vi "sub_DSP_main.vi"(8 "error in":errorcluster) -> (0 "error out":errorcluster)   [LabVIEW 2019]
uses:
  _ctrl/create-rw-close.ctl
  _ctrl/DSP_action.ctl
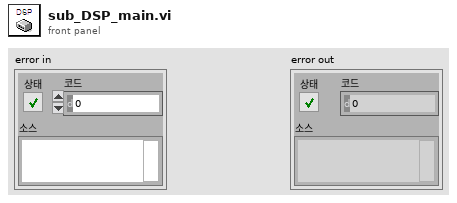
[diagram p1: front panel]
types:
  T1 = typedef "create-rw-close.ctl" = enum16{"create", "write", "read", "delete", "close"}
  T2 = typedef "DSP_action.ctl" = enum16{"False", "cont", "on", "off", "discont", "protection", "protection_seq", "preread", "level_seq", "level_m", "read", "stop", "exit"}
  T3 = typedef "DSP_action.ctl" = enum16{"False", "cont", "on", "off", "discont", "protection", "preread", "level", "read", "stop", "exit"}
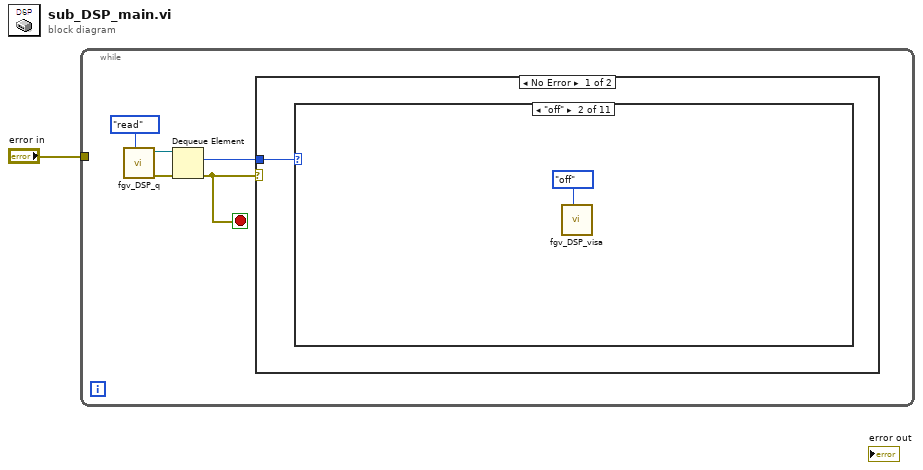
[diagram p0: block diagram]
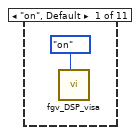
[diagram p2: hidden frame]
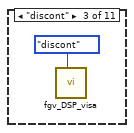
[diagram p3: hidden frame]
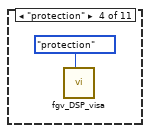
[diagram p4: hidden frame]
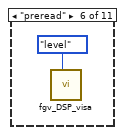
[diagram p6: hidden frame]
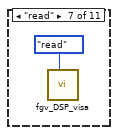
[diagram p7: hidden frame]
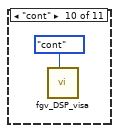
[diagram p10: hidden frame]
diagram:
  n1 = while {
    tunnel: "error in" -> [_]
    stop <- w2 stop-if-true
    n2 = call "fgv_DSP_q.vi"("cmd"=create-rw-close."read") -> ("error out"=w5:errorcluster, "queue out"=w4:refnum<queue>)  [unwired: 9 in]
    n3 = Dequeue Element(queue=w4, error in (no error)=w5) -> (element=w3:T2, error out=w2:errorcluster)  [unwired: 1 in, 2 out]
    n4 = case shown="No Error" w2 {
      tunnel: w3 -> [w7 _]
      frame No Error {
        n5 = case shown="\"off\"" w7 {
          frame "on", Default {
            n6 = call "fgv_DSP_visa.vi"("action"=DSP_action."on") -> ()  [unwired: 10 in, 1 out]
          }
          frame "off" {
            n7 = call "fgv_DSP_visa.vi"("action"=DSP_action."off") -> ()  [unwired: 10 in, 1 out]
          }
          frame "discont" {
            n8 = call "fgv_DSP_visa.vi"("action"=DSP_action."discont") -> ()  [unwired: 10 in, 1 out]
          }
          frame "protection" {
            n9 = call "fgv_DSP_visa.vi"("action"=DSP_action."protection") -> ()  [unwired: 10 in, 1 out]
          }
          frame "preread" {
          }
          frame "preread" {
            n10 = call "fgv_DSP_visa.vi"("action"=DSP_action."level") -> ()  [unwired: 10 in, 1 out]
          }
          frame "read" {
            n11 = call "fgv_DSP_visa.vi"("action"=DSP_action."read") -> ()  [unwired: 10 in, 1 out]
          }
          frame "stop" {
          }
          frame "exit" {
          }
          frame "cont" {
            n12 = call "fgv_DSP_visa.vi"("action"=DSP_action."cont") -> ()  [unwired: 10 in, 1 out]
          }
          frame "False" {
          }
        }
      }
      frame Error {
      }
    }
  }
